vi "niDTS WLAN UTIL Channel to Freq.vi"(6 "secondary factor":i32(ring)=1 items=["-1"=-1, "1"=1, "0"=0], 8 "error in":errorcluster, 9 "channel starting factor":dbl=10000.0, 10 "CH BW":T1, 11 "Channel":u32) -> (0 "error out":errorcluster, 2 "Center Frequency (GHz)":dbl, 3 "Center Frequency (Hz)":dbl)   [LabVIEW 2015, in "niDTS WLAN.lvlib"]
uses:
  niDTS WLAN.lvlib
  Includes/niDTS WLAN INC CH BW.ctl
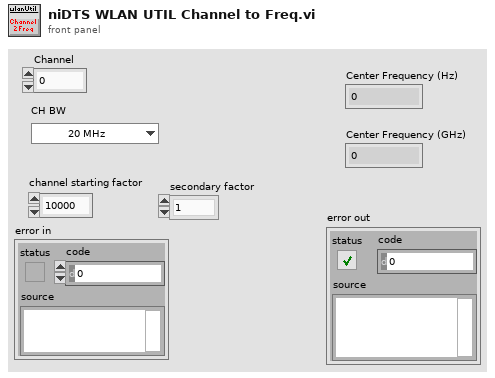
[diagram p1: front panel]
types:
  T1 = typedef "niDTS WLAN.lvlib/niDTS WLAN INC CH BW.ctl" = enum16{"20 MHz", "40 MHz", "80 MHz", "160 MHz"}
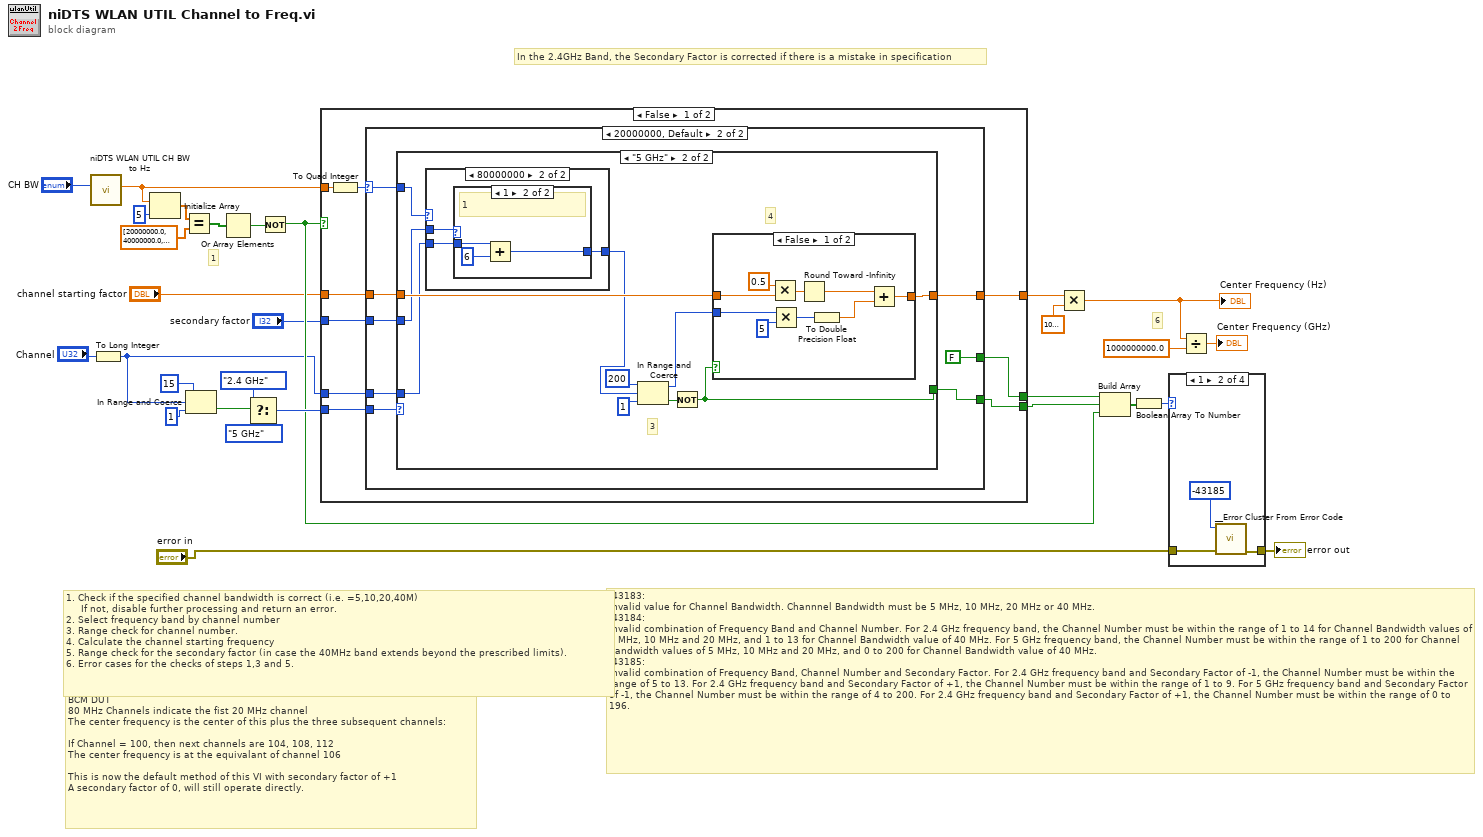
[diagram p0: block diagram]
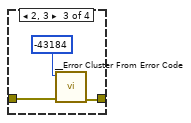
[diagram p3: hidden frame]
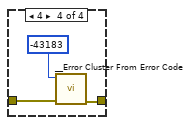
[diagram p4: hidden frame]
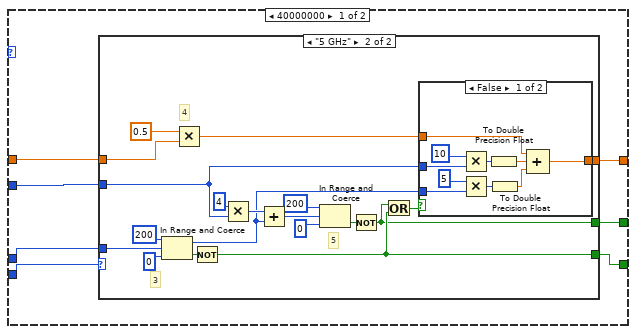
[diagram p5: hidden frame]
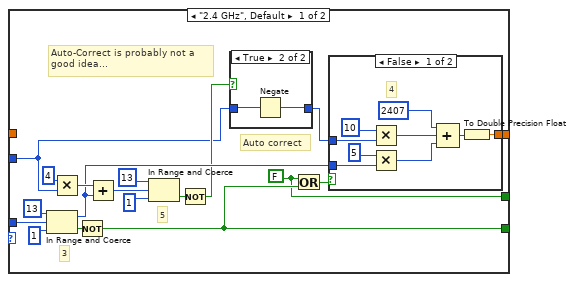
[diagram p6: hidden frame]
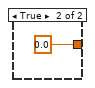
[diagram p8: hidden frame]
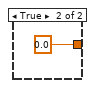
[diagram p9: hidden frame]
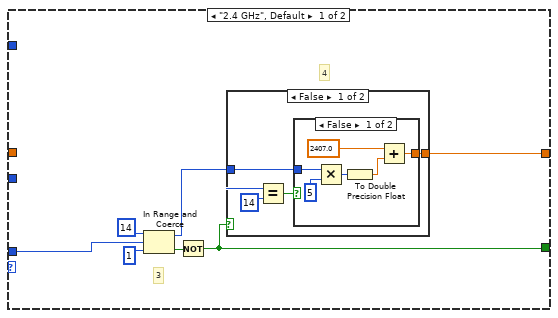
[diagram p10: hidden frame]
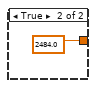
[diagram p11: hidden frame]
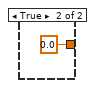
[diagram p12: hidden frame]
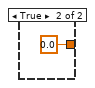
[diagram p15: hidden frame]
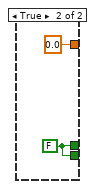
[diagram p16: hidden frame]
diagram:
  # "BCM DUT\n80 MHz Channels indicate the fist 20 MHz channel\nThe center frequency is the center of this plus the three subsequent channels:\n\nIf Channel = 100, then next channels are 104, 108, 112\nThe center frequency is at the equivalant of channel 106\n\nThis is now the default method of this VI with secondary factor of +1\nA secondary factor of 0, will still operate directly."
  # "In the 2.4GHz Band, the Secondary Factor is corrected if there is a mistake in specification"
  # "-43183:\nInvalid value for Channel Bandwidth. Channnel Bandwidth must be 5 MHz, 10 MHz, 20 MHz or 40 MHz.\n-43184:\nInvalid combination of Frequency Band and Channel Number. For 2.4 GHz frequency band, the Channel Number must be within the range of 1 to 14 for Channel Bandwidth values of 5 MHz, 10 MHz and 20 MHz, and 1 to 13 for Channel Bandwidth value of 40 MHz. For 5 GHz frequency band, the Channel Number must be within the range of 1 to 200 for Channel Bandwidth values of 5 MHz, 10 MHz and 20 MHz, and 0 to 200 for Channel Bandwidth value of 40 MHz.\n-43185:\nInvalid combination of Frequency Band, Channel Number and Secondary Factor. For 2.4 GHz frequency band and Secondary Factor of -1, the Channel Number must be within the range of 5 to 13. For 2.4 GHz frequency band and Secondary Factor of +1, the Channel Number must be within the range of 1 to 9. For 5 GHz frequency band and Secondary Factor of -1, the Channel Number must be within the range of 4 to 200. For 2.4 GHz frequency band and Secondary Factor of +1, the Channel Number must be within the range of 0 to 196."
  # "1. Check if the specified channel bandwidth is correct (i.e. =5,10,20,40M)\n     If not, disable further processing and return an error.\n2. Select frequency band by channel number \n3. Range check for channel number.\n4. Calculate the channel starting frequency\n5. Range check for the secondary factor (in case the 40MHz band extends beyond the prescribed limits). \n6. Error cases for the checks of steps 1,3 and 5."
  # "1"
  # "6"
  n1 = call "niDTS WLAN UTIL CH BW to Hz.vi"("CH BW"="CH BW") -> ("CH BW Hz"=w1:dbl)  [unwired: 10 in]
  n2 = To Long Integer(number="Channel") -> (32bit integer=w6:i32)
  n3 = Initialize Array(w1, 5 ("dimension size")) -> (w24:dbl[])
  n4 = Equal?(x=w24, y=dbl[] [20000000.0, 40000000.0, 80000000.0, 160000000.0, 80000000.0]) -> (x = y?=w22:bool[])
  n5 = In Range and Coerce(upper limit=u32 15 ("lower limit"), x=w6, lower limit=u32 1) -> (In Range?=w21:bool)  [unwired: 1 out]
  n6 = Or Array Elements(Boolean array=w22) -> (logical OR=w12:bool)
  n7 = Select(t=enum16{"2.4 GHz", "5 GHz"}."2.4 GHz" ("frequency band"), s=w21, f=enum16{"2.4 GHz", "5 GHz"}."5 GHz" ("frequency band")) -> (s? t:f=w18:enum16{"2.4 GHz", "5 GHz"})
  n8 = Not(x=w12) -> (.not. x?=w11:bool)
  n9 = case shown="False" w11 {
    tunnel: w18 -> [w38 _]
    tunnel: "channel starting factor" -> [w37 _]
    tunnel: w6 -> [w36 _]
    tunnel: "secondary factor" -> [w35 _]
    tunnel: [w34 0.0] -> w26
    tunnel: w1 -> [w32 _]
    tunnel: [w30 w163] -> w14
    tunnel: [w31 w163] -> w13
    frame False {
      n10 = To Quad Integer(1:w32) -> (0:w33:i64)
      n11 = case shown="20000000, Default" w33 {
        selector: w33 -> [_ w107]
        tunnel: w38 -> [w44 w114]
        tunnel: w37 -> [w45 w113]
        tunnel: [w41 w112] -> w34
        tunnel: w36 -> [w43 w111]
        tunnel: w35 -> [w42 w108]
        tunnel: [w40 w110] -> w31
        tunnel: [w39 FALSE] -> w30
        frame 40000000 {
          n12 = case shown="\"5 GHz\"" w44 {
            tunnel: w45 -> [_ w81]
            tunnel: [w61 w93] -> w41
            tunnel: w43 -> [w60 w92]
            tunnel: w42 -> [w47 w77]
            tunnel: [w50 w79] -> w40
            tunnel: [w49 w78] -> w39
            frame "2.4 GHz", Default {
              w49 = FALSE
              # "Auto-Correct is probably not a\ngood idea..."
              # "Auto correct"
              # "5"
              # "3"
              n13 = In Range and Coerce(upper limit=13, x=w60, lower limit=1) -> (coerced(x)=w52:i32, In Range?=w59:bool)
              n14 = Multiply(x=4, y=w47) -> (x*y=w54:i32)
              n15 = Not(x=w59) -> (.not. x?=w50:bool)
              n16 = Add(x=w54, y=w52) -> (x+y=w55:i32)
              n17 = In Range and Coerce(upper limit=13, x=w55, lower limit=1) -> (In Range?=w58:bool)  [unwired: 1 out]
              n18 = Not(x=w58) -> (.not. x?=w48:bool)
              n19 = case shown="True" w48 {
                tunnel: w47 -> [w64 w65]
                tunnel: [w64 w66] -> w46
                frame False {
                }
                frame True {
                  n20 = Negate(x=w65) -> (-x=w66:i32)
                }
              }
              n21 = Or(x=w49, y=w50) -> (x .or. y?=w51:bool)
              n22 = case shown="False" w51 {
                tunnel: [w74 0.0] -> w61
                tunnel: w52 -> [w68 _]
                tunnel: w46 -> [w67 _]
                frame False {
                  # "4"
                  n23 = Multiply(x=10 ("y"), y=w67) -> (x*y=w70:i32)
                  n24 = Multiply(x=5, y=w68) -> (x*y=w69:i32)
                  n25 = Compound Arithmetic op=ADD(2407 ("y"), w70, w69) -> (w72:i32)
                  n26 = To Double Precision Float(number=w72) -> (double precision float=w74:dbl)
                }
                frame True {
                }
              }
            }
            frame "5 GHz" {
              # "5"
              # "4"
              # "3"
              n27 = In Range and Coerce(upper limit=200, x=w92, lower limit=0) -> (coerced(x)=w84:i32, In Range?=w91:bool)
              n28 = Multiply(x=0.5, y=w81) -> (x*y=w82:dbl)
              n29 = Not(x=w91) -> (.not. x?=w79:bool)
              n30 = Multiply(x=4, y=w77) -> (x*y=w86:i32)
              n31 = Add(x=w86, y=w84) -> (x+y=w87:i32)
              n32 = In Range and Coerce(upper limit=200, x=w87, lower limit=0) -> (In Range?=w90:bool)  [unwired: 1 out]
              n33 = Not(x=w90) -> (.not. x?=w78:bool)
              n34 = Or(x=w78, y=w79) -> (x .or. y?=w83:bool)
              n35 = case shown="False" w83 {
                tunnel: [w98 0.0] -> w93
                tunnel: w84 -> [w101 _]
                tunnel: w77 -> [w100 _]
                tunnel: w82 -> [w99 _]
                frame False {
                  n36 = Multiply(x=10 ("y"), y=w100) -> (x*y=w103:i32)
                  n37 = Multiply(x=5, y=w101) -> (x*y=w102:i32)
                  n38 = To Double Precision Float(number=w103) -> (double precision float=w97:dbl)
                  n39 = To Double Precision Float(number=w102) -> (double precision float=w96:dbl)
                  n40 = Compound Arithmetic op=ADD(w99, w97, w96) -> (w98:dbl)
                }
                frame True {
                }
              }
            }
          }
        }
        frame 20000000, Default {
          n41 = case shown="\"5 GHz\"" w114 {
            tunnel: w113 -> [_ w144]
            tunnel: [w121 w143] -> w112
            tunnel: w111 -> [w119 w135]
            tunnel: [w115 w138] -> w110
            tunnel: w108 -> [_ w136]
            tunnel: w107 -> [_ w137]
            frame "2.4 GHz", Default {
              # "4"
              # "3"
              n42 = In Range and Coerce(upper limit=14, x=w119, lower limit=1) -> (coerced(x)=w120:i32, In Range?=w116:bool)
              n43 = Not(x=w116) -> (.not. x?=w115:bool)
              n44 = case shown="False" w115 {
                tunnel: [w123 0.0] -> w121
                tunnel: w120 -> [w122 _]
                frame False {
                  n45 = Equal?(x=w122, y=14) -> (x = y?=w124:bool)
                  n46 = case shown="False" w124 {
                    tunnel: w122 -> [w127 _]
                    tunnel: [w128 2484.0] -> w123
                    frame False {
                      n47 = Multiply(x=w127, y=5) -> (x*y=w130:i32)
                      n48 = To Double Precision Float(number=w130) -> (double precision float=w126:dbl)
                      n49 = Add(x=2407.0, y=w126) -> (x+y=w128:dbl)
                    }
                    frame True {
                    }
                  }
                }
                frame True {
                }
              }
            }
            frame "5 GHz" {
              # "4"
              # "3"
              n50 = case shown="80000000" w137 {
                tunnel: w136 -> [_ w148]
                tunnel: w135 -> [w145 w147]
                tunnel: [w145 w146] -> w134
                frame 0, Default {
                }
                frame 80000000 {
                  n51 = case shown="1" w148 {
                    tunnel: w147 -> [w149 w152]
                    tunnel: [w149 w150] -> w146
                    frame 0, Default {
                      # "-1 or 0"
                    }
                    frame 1 {
                      # "1"
                      n52 = Add(x=w152, y=6) -> (x+y=w150:i32)
                    }
                  }
                }
              }
              n53 = In Range and Coerce(upper limit=200, x=w134, lower limit=1) -> (coerced(x)=w140:i32, In Range?=w139:bool)
              n54 = Not(x=w139) -> (.not. x?=w138:bool)
              n55 = case shown="False" w138 {
                tunnel: w144 -> [w161 _]
                tunnel: [w155 0.0] -> w143
                tunnel: w140 -> [w154 _]
                frame False {
                  n56 = Multiply(x=0.5, y=w161) -> (x*y=w157:dbl)
                  n57 = Multiply(x=w154, y=5) -> (x*y=w158:i32)
                  n58 = Round Toward -Infinity(1:w157) -> (0:w156:dbl)
                  n59 = To Double Precision Float(number=w158) -> (double precision float=w153:dbl)
                  n60 = Add(x=w156, y=w153) -> (x+y=w155:dbl)
                }
                frame True {
                }
              }
            }
          }
        }
      }
    }
    frame True {
      w163 = FALSE
    }
  }
  n61 = Multiply(x=w26, y=1000000.0) -> (x*y=w4:dbl)
  "Center Frequency (Hz)" <- w4
  n62 = Build Array(w14, w13, w11) -> (w17:bool[])
  n63 = Boolean Array To Number(Boolean array=w17) -> (number=w16:u32)
  n64 = case shown="1" w16 {
    tunnel: "error in" -> [w165 w167 w170 w173]
    tunnel: [w165 w168 w171 w174] -> w8
    frame 0, Default {
    }
    frame 1 {
      n65 = call "__Error Cluster From Error Code.vi"("error in (no error)"=w167, "error code (0)"=-43185) -> ("error out"=w168:errorcluster)  [unwired: 1 in, 6 out]
    }
    frame 2, 3 {
      n66 = call "__Error Cluster From Error Code.vi"("error in (no error)"=w170, "error code (0)"=-43184) -> ("error out"=w171:errorcluster)  [unwired: 1 in, 6 out]
    }
    frame 4 {
      n67 = call "__Error Cluster From Error Code.vi"("error in (no error)"=w173, "error code (0)"=-43183) -> ("error out"=w174:errorcluster)  [unwired: 1 in, 6 out]
    }
  }
  "error out" <- w8
  n68 = Divide(x=w4, y=1000000000.0) -> (x/y=→"Center Frequency (GHz)":dbl)
